vi "SE FP hindbrain ACT.vi"(4 "MSpeed":dbl(slide) scale=0.0005..0.0025 scale format="%#.1g", 6 "Manual?":bool=TRUE, 7 "GPS?":bool=TRUE, 8 "error in":errorcluster, 9 "Act Com":T1, 10 "MHeading":dbl(slide) scale=0.0005..0.0025 scale format="%_1f", 11 "Current Boat Speed":dbl) -> (0 "error out":errorcluster, 1 "Speed":dbl min=-9.0 max=9.0 step=1.0, 2 "Desired \nRudder":dbl, 3 "Desired\nSpeed":dbl, 5 "Rudder":dbl min=-45.0 max=45.0 step=1.0)   [LabVIEW 2014]
doc: "This vi has two functions: it selects between manual and auto mode and it converts the incoming value into speed and rudder control values."
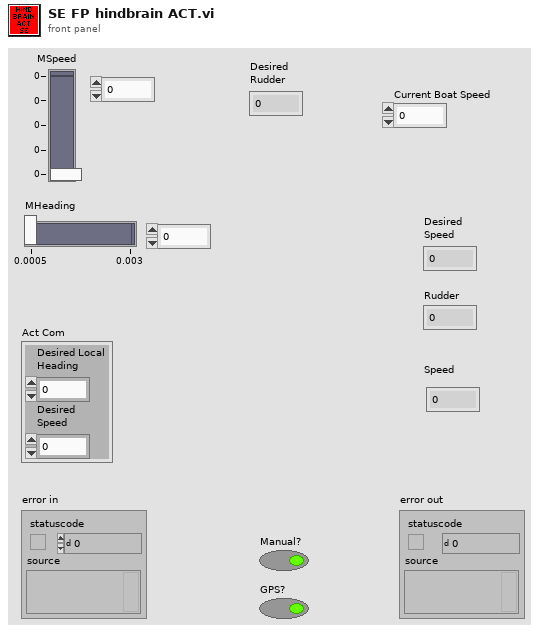
[diagram p1: front panel]
types:
  T1 = cluster{"Desired Local\nHeading":dbl, "Desired\nSpeed":dbl}
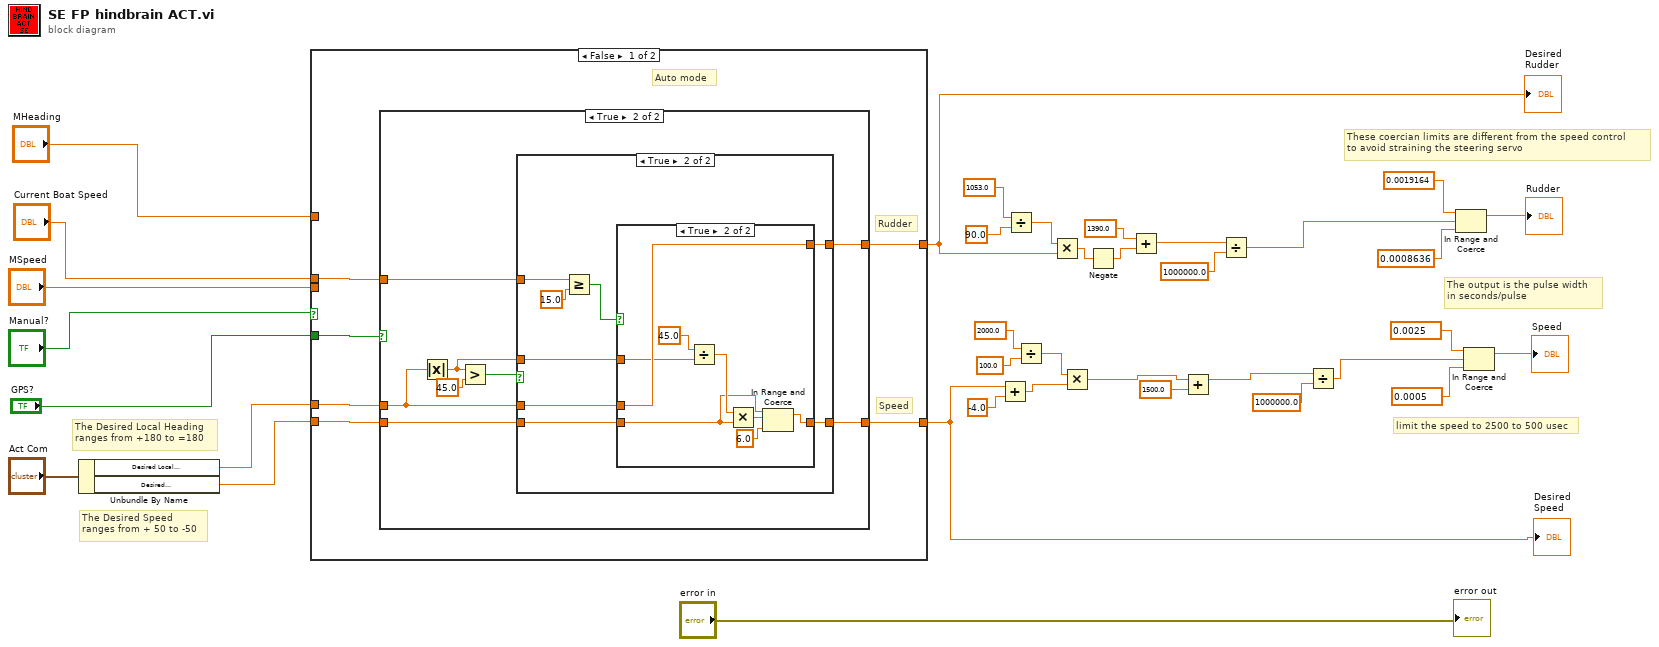
[diagram p0: block diagram]
diagram:
  # "These coercian limits are different from the speed control\nto avoid straining the steering servo"
  # "The output is the pulse width\nin seconds/pulse"
  # "The Desired Local Heading\nranges from +180 to =180"
  # "The Desired Speed\nranges from + 50 to -50"
  # "limit the speed to 2500 to 500 usec"
  n1 = Unbundle By Name("Act Com") -> ("Desired Local\nHeading"=w28:dbl, "Desired\nSpeed"=w27:dbl)
  n2 = case shown="False" "Manual?" {
    tunnel: w28 -> [w38 _]
    tunnel: [w41 w74] -> w2
    tunnel: w27 -> [w40 _]
    tunnel: [w39 w73] -> w5
    tunnel: "MHeading" -> [_ w74]
    tunnel: "MSpeed" -> [_ w73]
    tunnel: "Current Boat Speed" -> [w42 _]
    tunnel: "GPS?" -> [w37 _]
    frame False {
      # "Speed"
      # "Rudder"
      # "Auto mode"
      n3 = case shown="True" w37 {
        tunnel: w42 -> [_ w50]
        tunnel: [w44 w49] -> w41
        tunnel: w40 -> [w43 w48]
        tunnel: [w43 w47] -> w39
        tunnel: w38 -> [w44 w46]
        frame False {
        }
        frame True {
          n4 = Absolute Value(x=w46) -> (abs(x)=w45:dbl)
          n5 = Greater?(x=w45, y=45.0 ("x")) -> (0:w51:bool)
          n6 = case shown="True" w51 {
            tunnel: w50 -> [_ w62]
            tunnel: [w53 w57] -> w49
            tunnel: w48 -> [w54 w58]
            tunnel: [w54 w59] -> w47
            tunnel: w46 -> [w53 w56]
            tunnel: w45 -> [_ w55]
            frame False {
            }
            frame True {
              n7 = Greater Or Equal?(x=w62, y=15.0) -> (x >= y?=w60:bool)
              n8 = case shown="True" w60 {
                tunnel: [w64 w67] -> w59
                tunnel: w58 -> [w64 w66]
                tunnel: [w63 w72] -> w57
                tunnel: w56 -> [w63 w72]
                tunnel: w55 -> [_ w71]
                frame False {
                }
                frame True {
                  n9 = Divide(x=45.0, y=w71) -> (x/y=w70:dbl)
                  n10 = Multiply(x=w70, y=w66) -> (x*y=w68:dbl)
                  n11 = In Range and Coerce(upper limit=w66, x=w68, lower limit=6.0) -> (coerced(x)=w67:dbl)  [unwired: 1 out]
                }
              }
            }
          }
        }
      }
    }
    frame True {
      # "Manual mode"
    }
  }
  "Desired \nRudder" <- w2
  "Desired\nSpeed" <- w5
  n12 = Add(x=w5, y=-4.0) -> (x+y=w10:dbl)
  n13 = Divide(x=1053.0, y=90.0) -> (x/y=w21:dbl)
  n14 = Divide(x=2000.0, y=100.0) -> (x/y=w17:dbl)
  n15 = Multiply(x=w21, y=w2) -> (x*y=w7:dbl)
  n16 = Multiply(x=w17, y=w10) -> (x*y=w9:dbl)
  n17 = Negate(x=w7) -> (-x=w6:dbl)
  n18 = Add(x=1390.0, y=w6) -> (x+y=w15:dbl)
  n19 = Add(x=w9, y=1500.0) -> (x+y=w14:dbl)
  n20 = Divide(x=w15, y=1000000.0) -> (x/y=w3:dbl)
  n21 = Divide(x=w14, y=1000000.0) -> (x/y=w4:dbl)
  n22 = In Range and Coerce(upper limit=0.0019164 ("t"), x=w3, lower limit=0.0008636 ("t")) -> (coerced(x)=→"Rudder":dbl)  [unwired: 1 out]
  n23 = In Range and Coerce(upper limit=0.0025 ("t"), x=w4, lower limit=0.0005 ("t")) -> (coerced(x)=→"Speed":dbl)  [unwired: 1 out]
  "error out" <- "error in"
